vi "Untitled 6.vi"   [LabVIEW 2023]
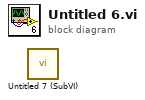
[diagram p0: block diagram]
diagram:
  n1 = call "Untitled 7 (SubVI).vi"() -> ()  [unwired: 10 in, 2 out]
